vi "TestSyncGrip.vi"() -> ()   [LabVIEW 2017]
uses:
  Projekt-RubikLibrary/ServoEnumControl.ctl
  <vilib>/myRIO/Common/Instrument Driver Framework/myRIO v1.0/UART/vis/myRIO v1.0 Close UART.vi
  <vilib>/myRIO/Common/Instrument Driver Framework/Utilities/vis/FPGA Ref Manager.vi
  <vilib>/myRIO/Common/Instrument Driver Framework/myRIO v1.0/myRIO v1.0 Reset FPGA.vi
  <vilib>/myRIO/Common/Instrument Driver Framework/myRIO v1.0/IRQ/vis/myRIO v1.0 IRQ Info FGV.vi
  <vilib>/myRIO/Common/Instrument Driver Framework/myRIO v1.0/IRQ/vis/myRIO v1.0 Timer IRQ Info FGV.vi
  <vilib>/myRIO/Common/Instrument Driver Framework/myRIO v1.0/IRQ/vis/myRIO v1.0 ISR Agent.vi
  Projekt-RubikLibrary/RubikLibraryRT.lvlib
  <vilib>/myRIO/Instrument Drivers/Utilities/Utilities.lvlib
  Projekt-RubikLibrary/RubikLibrary.lvlib
panel:
  in  "Servo 3":T1=enum."Right Servo"
  in  "NoWait 3":bool=TRUE
  in  "stop":bool
  in  "NoWait 2":bool=TRUE
  in  "NoWait 1":bool=TRUE
  in  "Grip closed (in)":bool
  in  "Servo 2":T1=enum."Front Servo"
  in  "Servo 1":T1
  # "Test Synchronous Behaviour of 3 Grip Servos\n\n\"Synchronous\" means that VI(software) does not\nwait (default 500ms). So you will observe\nsynchronous behaviour: all three grips will move\nsynchronously.\n\nThe VI does not wait for completion of grip.\n\nYou will call this asynchronous execution of the software!\n\n\"NoWait==T\" means grips execute in parallel\n\"NoWait==F\" shows one grip after the other."
  # "Initial postion:\nAll three servos open \nand at 0° (vertical)!"
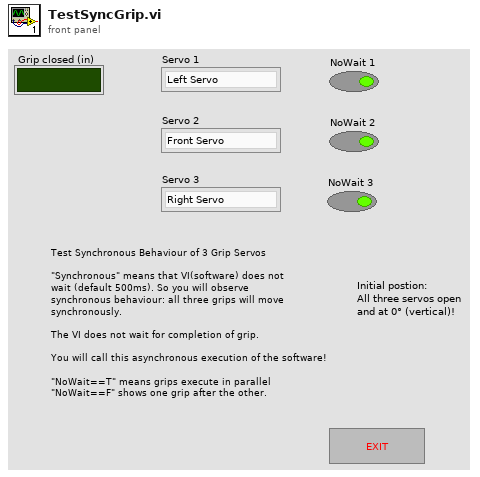
[diagram p1: front panel]
types:
  T1 = typedef "RubikLibrary.lvlib/ServoEnumControl.ctl" = enum16{"Left Servo", "Front Servo", "Right Servo"}
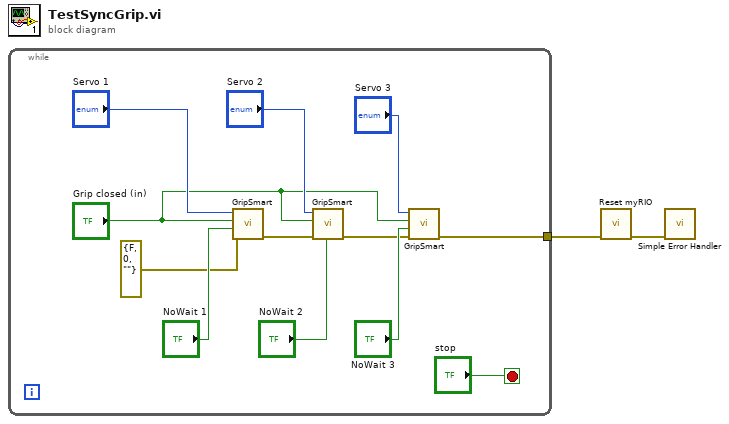
[diagram p0: block diagram]
diagram:
  n1 = while {
    tunnel: [w3] -> w1
    stop <- "stop" stop-if-true
    n2 = call "GripSmart.vi"("error in"=errorcluster {"status"=FALSE, "code"=0, "source"=""}, "NoWait"="NoWait 1", "Grip closed (in)"="Grip closed (in)", "Servo"="Servo 1") -> ("error out"=w14:errorcluster)  [unwired: 6 in, 1 out]
    n3 = call "GripSmart.vi"("error in"=w14, "NoWait"="NoWait 2", "Grip closed (in)"="Grip closed (in)", "Servo"="Servo 2") -> ("error out"=w6:errorcluster)  [unwired: 6 in, 1 out]
    n4 = call "GripSmart.vi"("error in"=w6, "NoWait"="NoWait 3", "Grip closed (in)"="Grip closed (in)", "Servo"="Servo 3") -> ("error out"=w3:errorcluster)  [unwired: 6 in, 1 out]
  }
  n5 = call <vilib>:"Reset myRIO.vi"("error in (no error)"=w1) -> ("error out"=w2:errorcluster)  [unwired: 10 in]
  n6 = call <vilib>:"Simple Error Handler.vi"("error in (no error)"=w2) -> ()  [unwired: 4 in, 5 out]
